vi "John's Video Viewer.vi"() -> ()   [LabVIEW 2018]
uses:
  John's Video Viewer Status STYP.ctl
  Classes/Video File/Video File.lvclass
  <vilib>/vision/Image Controls.llb/IMAQ Image.ctl
  Classes/Video Frame/Video Frame.lvclass
  Classes/Roughness Averager/Roughness Averager.lvclass
  Classes/Pointcloud/Pointcloud.lvclass
  <userlib>/Jet Engineering/JET_QSM/Code/Private/JET_QSM_InvalidOption STYP.ctl
  Classes/Video File/Video File.lvclass/Video File.ctl
  <userlib>/Jet Engineering/JET_QSM/Code/Private/JET_QSM - Add State [String API].vi
  Classes/Video File/Read Frame Data.vi
  Classes/ROIed Video Frame/ROIed Video Frame.lvclass
  C:/Users/aaron.jencks/Documents/GitHub/emerson_seed_object_detection/LabVIEW/Projects/Paul's Video Viewer/Classes/Video Frame/Video Frame.lvclass
  <vilib>/Utility/error.llb/Trim Whitespace.vi
  <vilib>/Utility/error.llb/Error Cluster From Error Code.vi
panel:
  out "width, X":i32=1280
  out "height, Y":i32=720
  out "3D Picture":refnum<vi>(3d-picture)
  out "Standard Deviation":dbl[](graph)
  in  "stop":bool
  in  "FPS":i32(slide) scale=10.0..90.0
  out "Roughness":dbl[](graph)
  out "Depth":T1(plugin-control)
  out "RGB":T1(plugin-control)
  in  "Video File":path
  out "Recent states before Error (with tick counts) 2":string="0.167 sec ago: VI Initialize\n0.167 sec ago: Window Open\n0.110 sec ago: Control Update\n0.110 sec ago: Indicator Update\n0.000 sec ago: Error Handler\r\n"
  out "error out":errorcluster
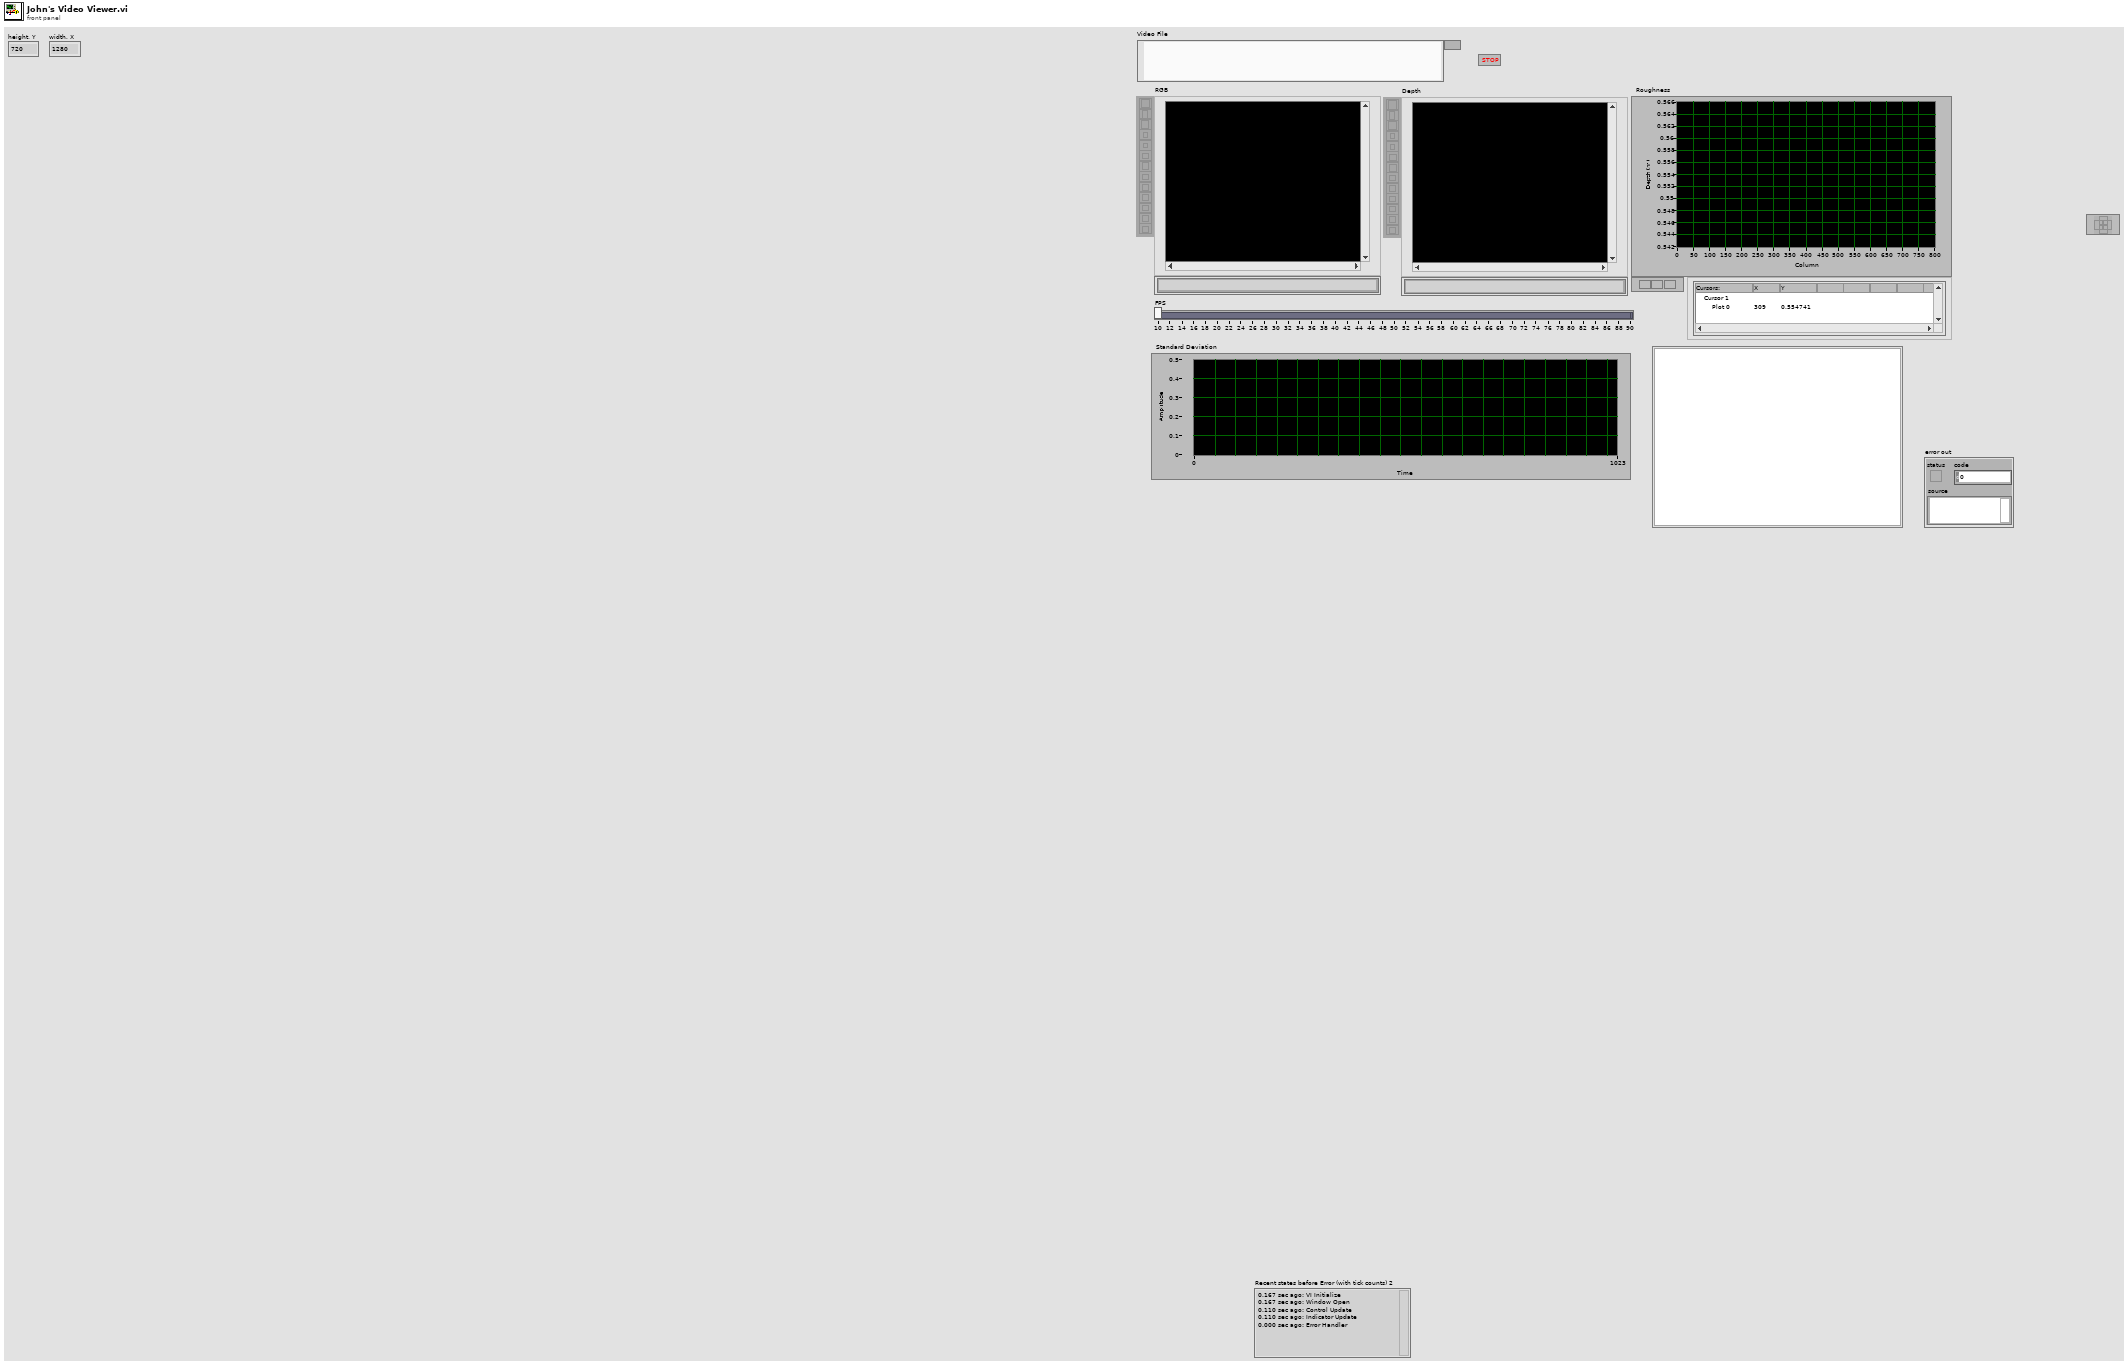
[diagram p1: front panel]
types:
  T1 = typedef "IMAQ Image.ctl" = refnum<image>
  T2 = typedef "John's Video Viewer Status STYP.ctl" = cluster{"VI":cluster{"error":errorcluster, "isExiting?":bool}, "UserLoggedIn?":bool, "RGB File":refnum<class "Video File.lvclass">, "Depth File":refnum<class "Video File.lvclass">, "RGB Image":T1, "Depth Image":T1, "RGB Frame":refnum<class "Video Frame.lvclass">, "Depth Frame":refnum<class "Video Frame.lvclass">, "FPS":i32, "History Average":refnum<queue>, "Standard Deviation":refnum<queue>, "Averager":refnum<class "Roughness Averager.lvclass">, "Pointcloud":refnum<class "Pointcloud.lvclass">}
  T3 = typedef "JET_QSM_InvalidOption STYP.ctl" = enum16{"Ignore", "Dialog", "Error"}
  T4 = typedef "JET_QSM_Refnum STYP.ctl" = cluster{"state":cluster{"queue":refnum<queue>, "idle":string, "error":string, "STOP":string}, "debug":cluster{"enabled?":bool, "queue":refnum<queue>}, "Invalid.option":T3, "QSM.Name":string}
  T5 = enum32{"invalid app kind", "Development System", "Run Time System", "Student Edition", "Embedded LabVIEW", "Evaluation", "Custom"}
  T6 = typedef "JET_QSM_Element STYP.ctl" = cluster{"state":string, "data":variant, "comment":string}
  T7 = cluster{"Width":u32, "Height":u32, "Frames Per Second":u32, "Codec":string, "Has Data":bool}
  T8 = cluster{"Global Rectangle":i32[], "Contours":cluster{"Contour Type":u32, "ROI Type":u32, "Points":i32[]}[]}
  T9 = cluster{"Normal":cluster{"Averages":cluster{"Average":dbl, "RMS":dbl, "Absolute Mean Deviation":dbl}, "Global Heuristics":cluster{"Max":dbl, "Min":dbl, "Max Peak-to-Peak":dbl}, "Skewdness":dbl, "Kurtosis":dbl, "RzDIN":dbl, "RzJIS":dbl}, "Slope Parameters":cluster{"Rdq":dbl, "Rda":dbl}, "Areal Roughness":cluster{"Peak Density":dbl}}
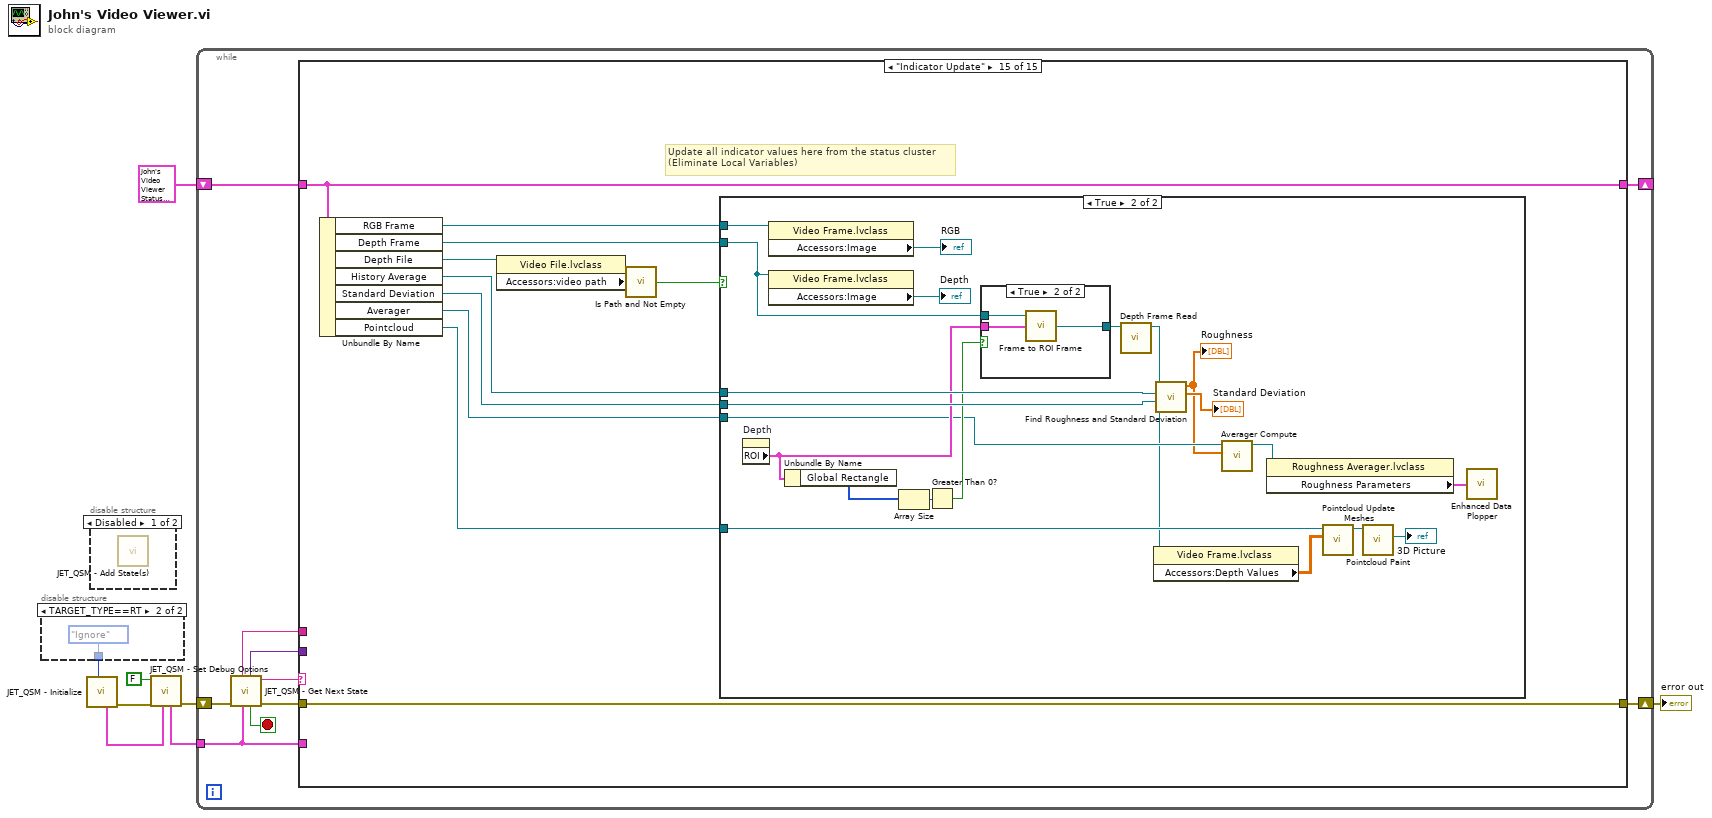
[diagram p0: block diagram]
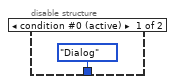
[diagram p2: hidden frame]
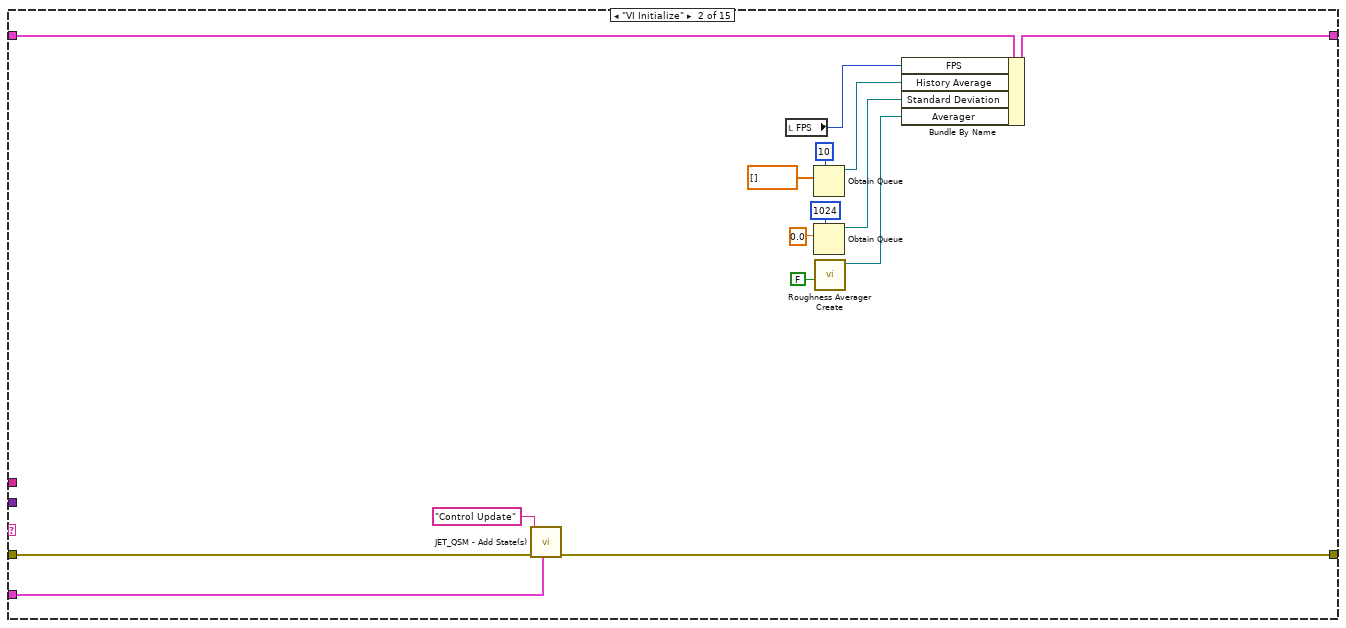
[diagram p5: hidden frame]
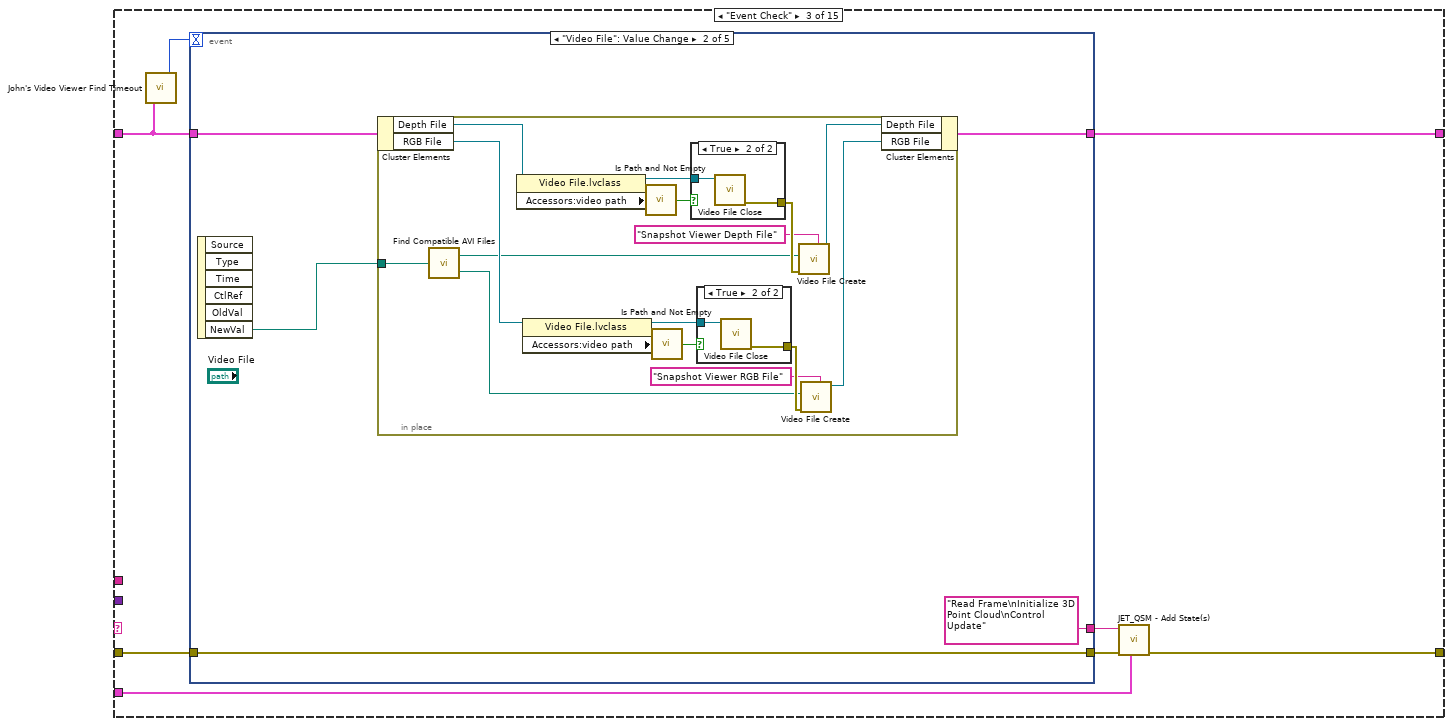
[diagram p6: hidden frame]
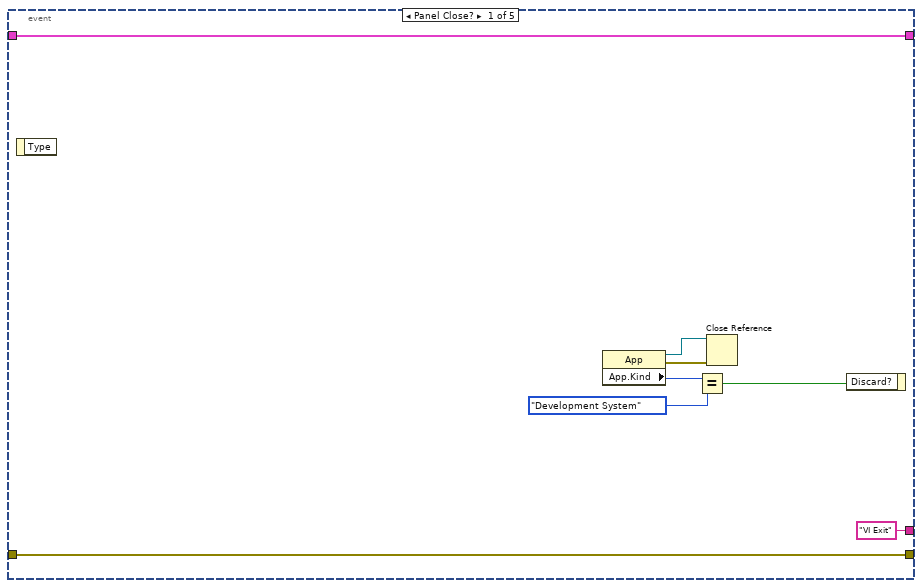
[diagram p7: hidden frame]
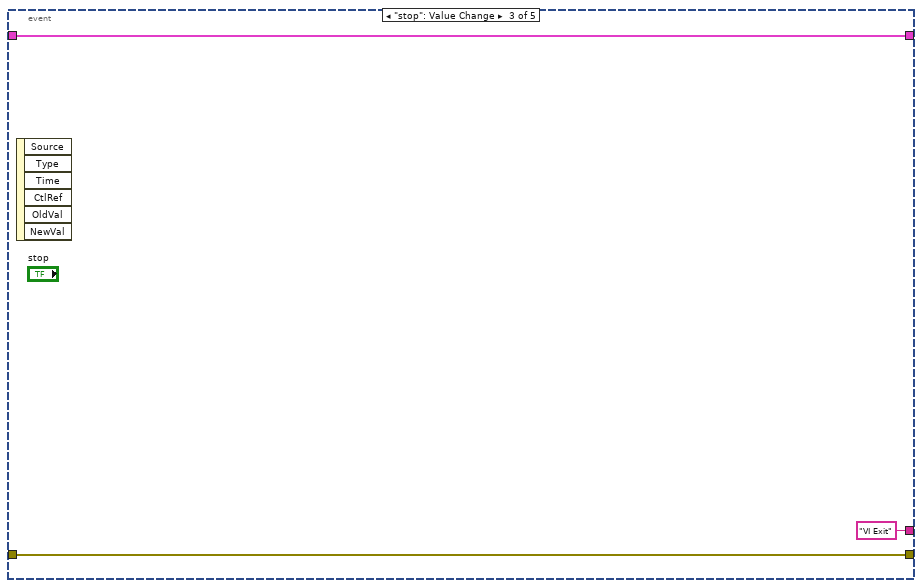
[diagram p10: hidden frame]
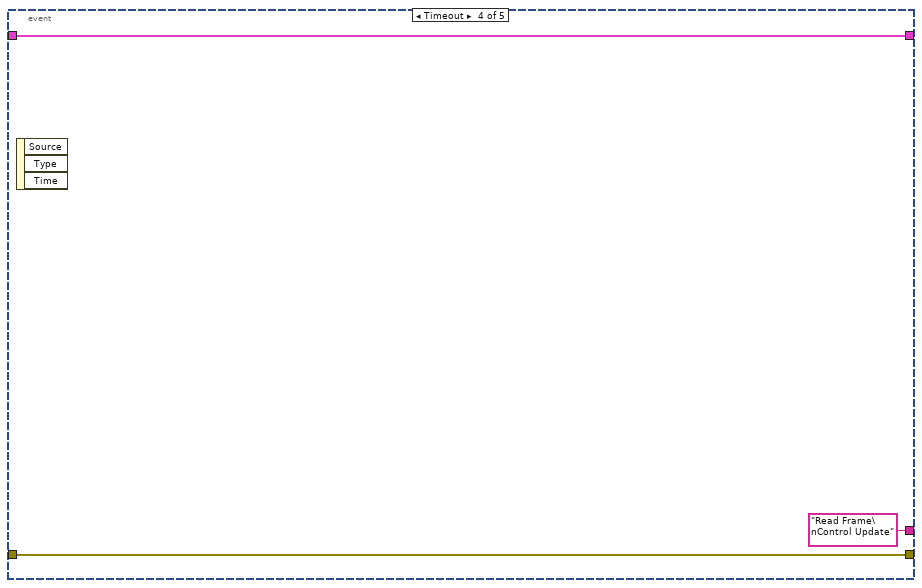
[diagram p11: hidden frame]
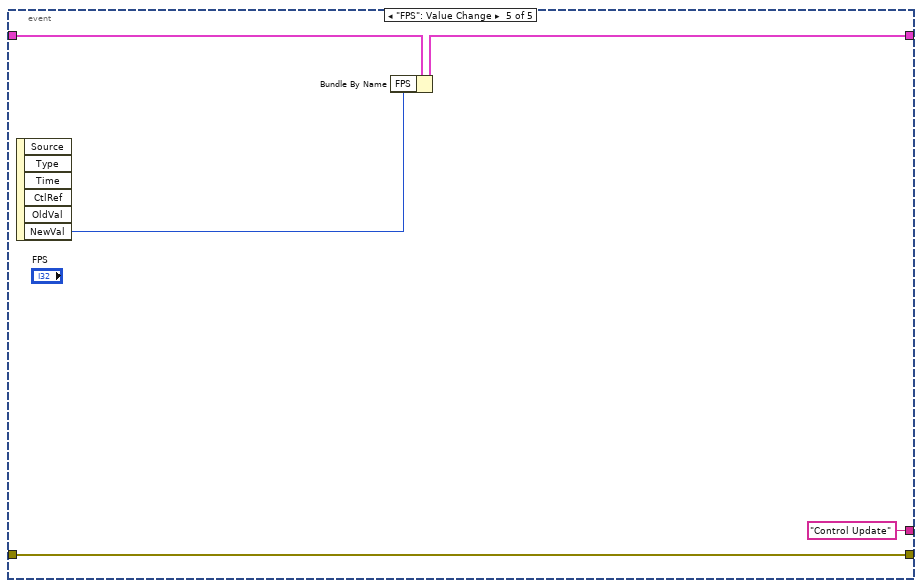
[diagram p12: hidden frame]
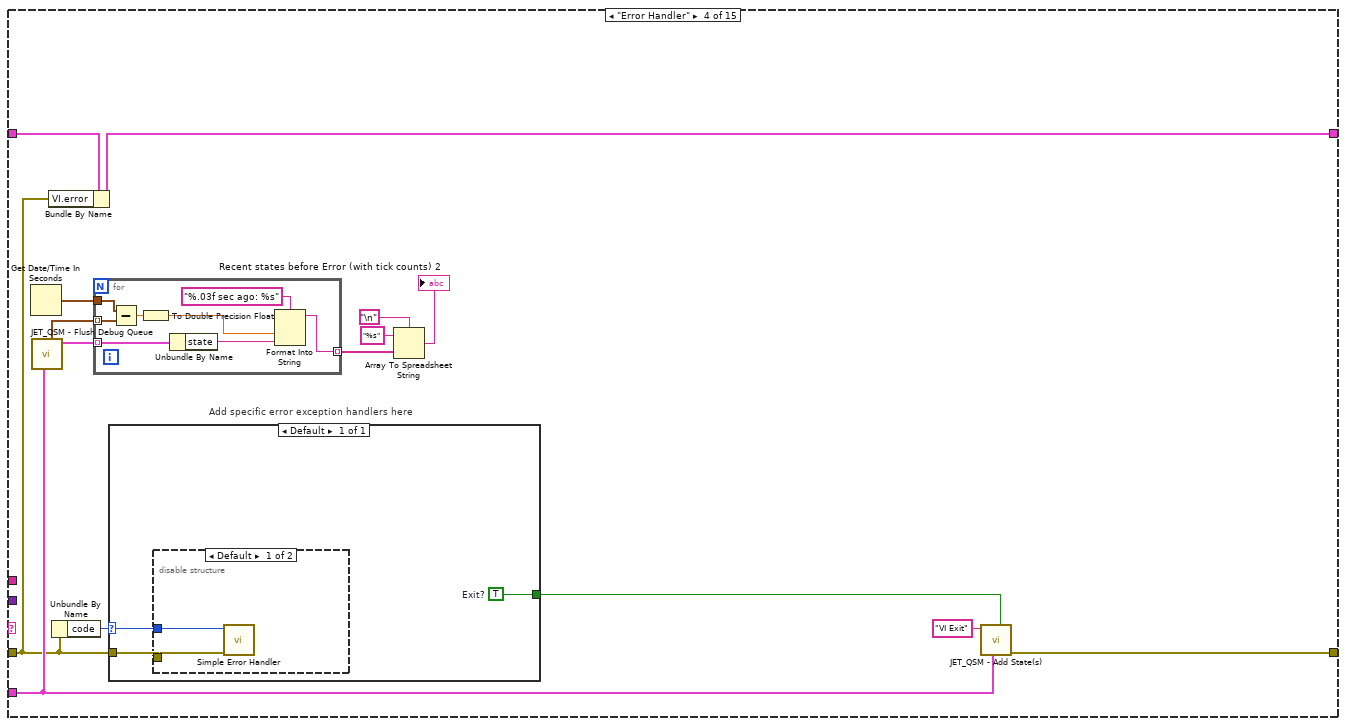
[diagram p13: hidden frame]
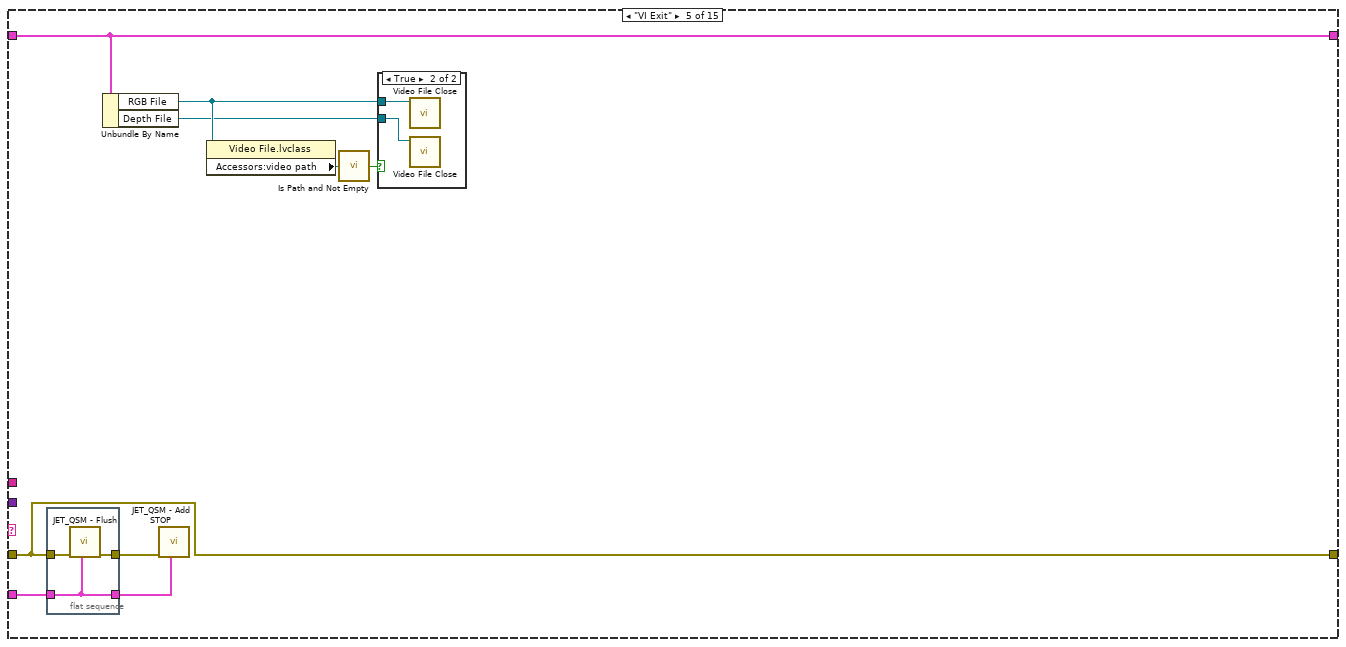
[diagram p15: hidden frame]
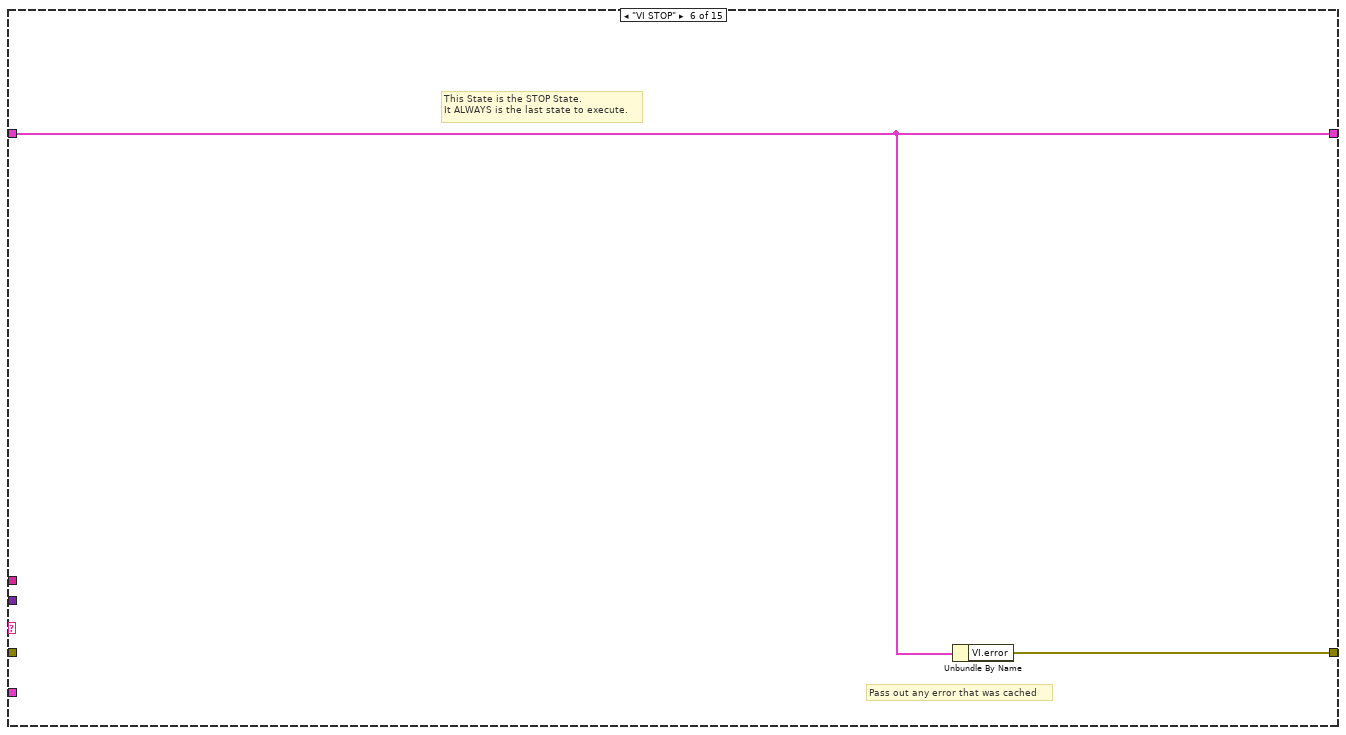
[diagram p17: hidden frame]
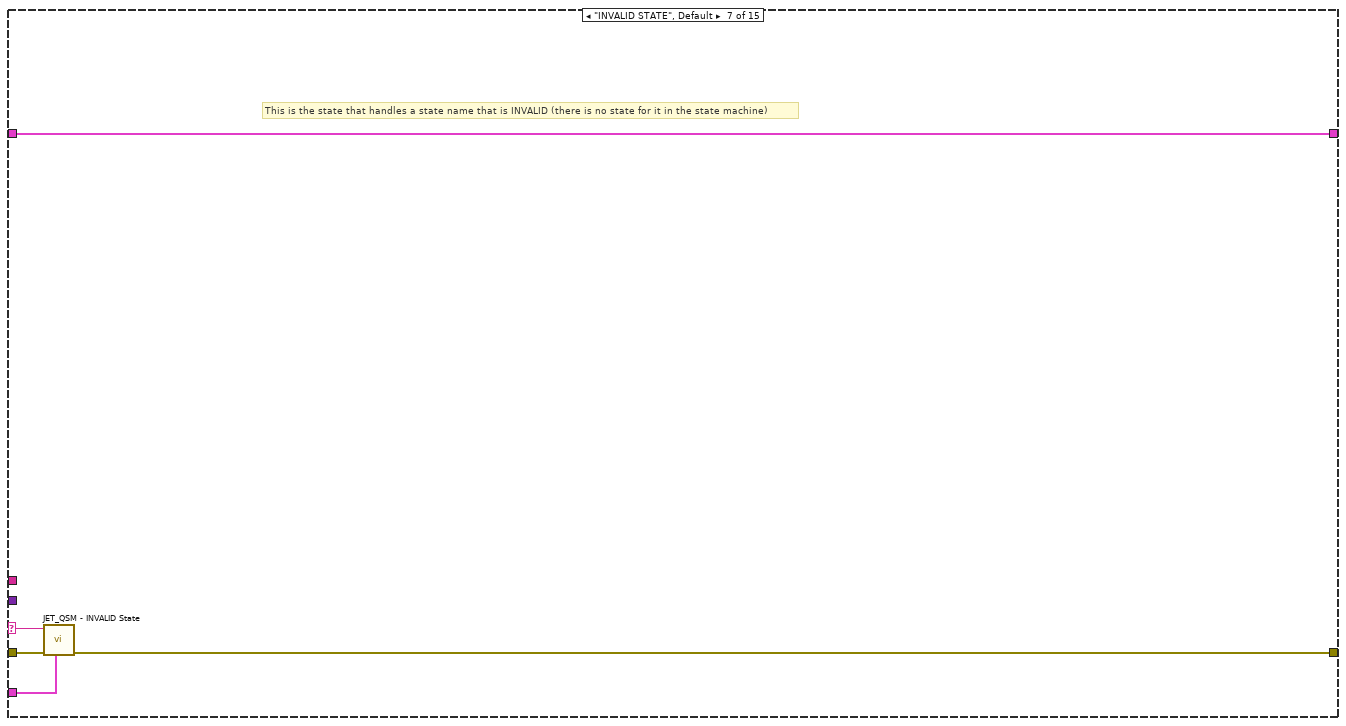
[diagram p18: hidden frame]
diagram:
  n1 = disable-structure shown="TARGET_TYPE==RT" {
    disable-tunnel: [JET_QSM_InvalidOption_STYP."Dialog" ("invalid state action (Dialog)") JET_QSM_InvalidOption_STYP."Ignore" ("invalid state action (Dialog)")] -> w8
    frame condition #0 (active) {
    }
    frame condition #1 {
    }
  }
  n2 = call <userlib>:"JET_QSM - Initialize.vi"("invalid state action (Dialog)"=w8) -> ("error out"=w1:errorcluster, "Jet_QSM refnum"=w4:T4)  [unwired: 9 in]
  n3 = disable-structure shown="Disabled" {
    frame Disabled {
      n4 = call-poly <userlib>:"JET_QSM - Add State(s).vi"() -> ()  [unwired: 11 in, 1 out]
    }
    frame Enabled {
    }
  }
  n5 = call <userlib>:"JET_QSM - Set Debug Options.vi"("Jet_QSM refnum"=w4, "error in (no error)"=w1, "debug.enabled? (F)"=FALSE) -> ("error out"=w2:errorcluster, "Jet_QSM ref"=w3:T4)  [unwired: 7 in]
  n6 = while {
    tunnel: w3 -> [w16]
    shift-right: [w14] -> _
    shift-left: T2 {"VI"={"error"={"status"=FALSE, "code"=0, "source"=""}, "isExiting?"=FALSE}, "UserLoggedIn?"=FALSE, "RGB File"=refnum, "Depth File"=refnum, "RGB Image"=refnum, "Depth Image"=refnum, "RGB Frame"=refnum, "Depth Frame"=refnum, "FPS"=0, "History Average"=refnum, "Standard Deviation"=refnum, "Averager"=refnum, "Pointcloud"=refnum} ("Status") -> [w15]
    shift-right: [w13] -> w7
    shift-left: w2 -> [w20]
    stop <- w17 stop-if-true
    n7 = call <userlib>:"JET_QSM - Get Next State.vi"("Jet_QSM refnum"=w16, "error in (no error)"=w20) -> ("error out"=w19:errorcluster, "state"=w18:string, "Stop Loop?"=w17:bool, "state data"=w12:variant, "state comment"=w11:string)  [unwired: 5 in]
    n8 = case shown="\"Indicator Update\"" w18 {
      selector: w18 -> [_ _ _ _ _ _ w137 _ _ _ _ _ _ _ _]
      tunnel: w19 -> [w21 w37 w45 w92 w127 _ w138 w140 w142 w144 w153 w156 w181 w188 w201]
      tunnel: w16 -> [_ w35 w44 w97 w125 _ w136 _ _ _ _ _ _ w189 _]
      tunnel: w15 -> [w22 w33 w38 w93 w123 w133 w139 w141 w143 w145 w150 w155 w182 w186 w200]
      tunnel: [w22 w32 w40 w91 w123 w133 w139 w141 w143 w145 w151 w154 w182 w186 w200] -> w14
      tunnel: [w21 w36 w42 w98 w127 w134 w135 w140 w142 w144 w153 w156 w181 w187 w201] -> w13
      tunnel: w12 -> [_ _ _ _ _ _ _ _ _ _ _ _ _ _ _]
      tunnel: w11 -> [_ _ _ _ _ _ _ _ _ _ _ _ _ _ _]
      frame "------ Standard States ------" {
        # "Standard States are required states for a JET_QSM State Machine\n\nTheir names may be changed; use the Initialize function to specify the new names"
        # "This is a section header; the state is never expected to execute"
      }
      frame "VI Initialize" {
        n9 = call-poly <userlib>:"JET_QSM - Add State(s).vi"("Jet_QSM refnum"=w35, "error in (no error)"=w37, "state(s)"="Control Update") -> ("error out"=w36:errorcluster)  [unwired: 8 in]
        n10 = local read "FPS"() -> (w31:i32)
        n11 = Obtain Queue(max queue size (-1, unlimited)=10, element data type=dbl[] []) -> (queue out=w29:refnum<queue>)  [unwired: 3 in, 2 out]
        n12 = Obtain Queue(max queue size (-1, unlimited)=1024, element data type=0.0) -> (queue out=w27:refnum<queue>)  [unwired: 3 in, 2 out]
        n13 = call "Roughness Averager Create.vi"("Full? (T)"=FALSE) -> ("Roughness Averager out"=w23:refnum<class "Roughness Averager.lvclass">)  [unwired: 9 in, 1 out]
        n14 = Bundle By Name(cluster=w33, "FPS"=w31, "History Average"=w29, "Standard Deviation"=w27, "Averager"=w23) -> (w32:T2)
      }
      frame "Event Check" {
        n15 = call "John's Video Viewer Find Timeout.vi"("Status"=w38) -> ("Timeout"=w39:i32)
        n16 = event shown="[1] \"Video File\": Value Change" {
          selector: _ -> [_ _ _ _ _]
          dyn-events: _ -> [_ _ _ _ _]
          timeout: w39 -> [_ _ _ _ _]
          tunnel: w45 -> [w47 w55 w81 w85 w90]
          tunnel: ["VI Exit" ("state(s)") "Read Frame\nInitialize 3D Point Cloud\nControl Update" ("state(s)") "VI Exit" ("state(s)") "Read Frame\nControl Update" ("state(s)") "Control Update" ("state(s)")] -> w43
          tunnel: [w47 w55 w81 w85 w90] -> w41
          tunnel: w38 -> [w46 w58 w82 w83 w88]
          tunnel: [w46 w57 w82 w83 w86] -> w40
          event Panel Close? {
            n17 = event-data() -> ()  [unwired: 1 in, 1 out]
            n18 = property class="App"() -> (reference out=w49:refnum<vi>, error out=w50:errorcluster, "App.Kind"=w53:T5)  [unwired: 2 in]
            n19 = Equal?(x=w53, y=T5."Development System") -> (x = y?=w51:bool)
            n20 = Close Reference(reference=w49, error in (no error)=w50) -> ()  [unwired: 1 out]
            n21 = event-data("Discard?"=w51) -> ()  [unwired: 1 in, 1 out]
          }
          event "Video File": Value Change {
            n22 = event-data() -> ("NewVal"=w56:path)  [unwired: 1 in, 5 out]
            n23 = in-place {
              in-place-border: w56 -> [w61]
              n24 = in-place-cluster #1(w58) -> ("Depth File"=w75:refnum<class "Video File.lvclass">, "RGB File"=w68:refnum<class "Video File.lvclass">)
              n25 = call "Find Compatible AVI Files.vi"("Video Path"=w61) -> ("RGB Path"=w59:path, "Depth Path"=w60:path)  [unwired: 2 in]
              n26 = property class="Video File.lvclass"(reference=w75) -> (reference out=w72:refnum<class "Video File.lvclass">, "Accessors:video path"=w74:path)  [unwired: 1 in, 1 out]
              n27 = property class="Video File.lvclass"(reference=w68) -> (reference out=w66:refnum<class "Video File.lvclass">, "Accessors:video path"=w67:path)  [unwired: 1 in, 1 out]
              n28 = call <vilib>:"Is Path and Not Empty.vi"("path"=w74) -> ("Is Path and Not Empty?"=w73:bool)  [unwired: 4 in]
              n29 = call <vilib>:"Is Path and Not Empty.vi"("path"=w67) -> ("Is Path and Not Empty?"=w65:bool)  [unwired: 4 in]
              n30 = case shown="True" w73 {
                tunnel: w72 -> [_ w79]
                tunnel: [_ w78] -> w70
                frame False {
                }
                frame True {
                  n31 = call-dynamic "Video File Close.vi"("Video File in"=w79) -> ("error out"=w78:errorcluster)  [unwired: 9 in, 1 out]
                }
              }
              n32 = case shown="True" w65 {
                tunnel: w66 -> [_ w77]
                tunnel: [_ w76] -> w64
                frame False {
                }
                frame True {
                  n33 = call-dynamic "Video File Close.vi"("Video File in"=w77) -> ("error out"=w76:errorcluster)  [unwired: 9 in, 1 out]
                }
              }
              n34 = call "Video File Create.vi"("Identifier"="Snapshot Viewer Depth File", "error in (no error)"=w70, "Video Path (\"\")"=w60) -> ("Video File out"=w71:refnum<class "Video File.lvclass">)  [unwired: 7 in, 1 out]
              n35 = call "Video File Create.vi"("Identifier"="Snapshot Viewer RGB File", "error in (no error)"=w64, "Video Path (\"\")"=w59) -> ("Video File out"=w62:refnum<class "Video File.lvclass">)  [unwired: 7 in, 1 out]
              n36 = in-place-cluster #1("Depth File"=w71, "RGB File"=w62) -> (w57:T2)
            }
          }
          event "stop": Value Change {
            n37 = event-data() -> ()  [unwired: 1 in, 6 out]
          }
          event Timeout {
            n38 = event-data() -> ()  [unwired: 1 in, 3 out]
          }
          event "FPS": Value Change {
            n39 = event-data() -> ("NewVal"=w87:i32)  [unwired: 1 in, 5 out]
            n40 = Bundle By Name(cluster=w88, "FPS"=w87) -> (w86:T2)
          }
        }
        n41 = call-poly <userlib>:"JET_QSM - Add State(s).vi"("Jet_QSM refnum"=w44, "error in (no error)"=w41, "state(s)"=w43) -> ("error out"=w42:errorcluster)  [unwired: 8 in]
      }
      frame "Error Handler" {
        # "Add specific error exception handlers here"
        n42 = Get Date/Time In Seconds() -> (seconds since 1Jan1904=w101:timestamp)
        n43 = call <userlib>:"JET_QSM - Flush Debug Queue.vi"("Jet_QSM refnum"=w97) -> ("QSM Elements"=w99:T6[], "Timestamps"=w100:timestamp[])  [unwired: 8 in, 1 out]
        n44 = Bundle By Name(cluster=w93, "VI.error"=w92) -> (w91:T2)
        n45 = Unbundle By Name(w92) -> ("code"=w94:i32)
        n46 = for {
          tunnel: w99 -> [w113] mode=indexing
          tunnel: [w111] -> w103 mode=indexing
          tunnel: w101 -> [w108]
          tunnel: w100 -> [w109] mode=indexing
          n47 = Subtract(x=w108, y=w109) -> (x-y=w107:dbl)
          n48 = To Double Precision Float(number=w107) -> (double precision float=w106:dbl)
          n49 = Unbundle By Name(w113) -> ("state"=w112:string)
          n50 = Format Into String(format string="%.03f sec ago: %s", w106, w112) -> (resulting string=w111:string)  [unwired: 2 in, 1 out]
        }
        n51 = case shown="Default" w94 {
          selector: w94 -> [w115]
          tunnel: [w116] -> w95
          tunnel: w92 -> [w114]
          frame Default {
            w116 = TRUE  # Exit?
            n52 = disable-structure shown="Default" {
              disable-tunnel: w115 -> [w118 _]
              disable-tunnel: w114 -> [w117 _]
              frame condition #0 (active) {
                n53 = call <vilib>:"Simple Error Handler.vi"("error code (no error:0)"=w118, "error in (no error)"=w117) -> ()  [unwired: 3 in, 5 out]
              }
              frame condition #1 {
              }
            }
          }
        }
        n54 = Array To Spreadsheet String(delimiter (Tab)="\n", array=w103, 3:"%s" ("format string")) -> (spreadsheet string=→"Recent states before Error (with tick counts) 2":string)
        n55 = call-poly <userlib>:"JET_QSM - Add State(s).vi"("act? (T)"=w95, "Jet_QSM refnum"=w97, "state(s)"="VI Exit") -> ("error out"=w98:errorcluster)  [unwired: 8 in]
      }
      frame "VI Exit" {
        n56 = flat-sequence {
          tunnel: w127 -> [w132]
          tunnel: [w131] -> w126
          tunnel: w125 -> [w130]
          tunnel: [w130] -> w124
          frame #0 {
            n57 = call <userlib>:"JET_QSM - Flush.vi"("Jet_QSM ref"=w130, "error in (no error)"=w132) -> ("error out"=w131:errorcluster)  [unwired: 8 in, 1 out]
          }
        }
        n58 = Unbundle By Name(w123) -> ("RGB File"=w120:refnum<class "Video File.lvclass">, "Depth File"=w119:refnum<class "Video File.lvclass">)
        n59 = call <userlib>:"JET_QSM - Add STOP.vi"("Jet_QSM refnum"=w124, "error in (no error)"=w126) -> ()  [unwired: 9 in, 1 out]
        n60 = property class="Video File.lvclass"(reference=w120) -> ("Accessors:video path"=w122:path)  [unwired: 1 in, 2 out]
        n61 = call <vilib>:"Is Path and Not Empty.vi"("path"=w122) -> ("Is Path and Not Empty?"=w121:bool)  [unwired: 4 in]
        n62 = case shown="True" w121 {
          tunnel: w120 -> [_ w129]
          tunnel: w119 -> [_ w128]
          frame False {
          }
          frame True {
            n63 = call-dynamic "Video File Close.vi"("Video File in"=w129) -> ()  [unwired: 9 in, 2 out]
            n64 = call-dynamic "Video File Close.vi"("Video File in"=w128) -> ()  [unwired: 9 in, 2 out]
          }
        }
      }
      frame "VI STOP" {
        # "Pass out any error that was cached"
        # "This State is the STOP State.\nIt ALWAYS is the last state to execute."
        n65 = Unbundle By Name(w133) -> ("VI.error"=w134:errorcluster)
      }
      frame "INVALID STATE", Default {
        # "This is the state that handles a state name that is INVALID (there is no state for it in the state machine)"
        n66 = call <userlib>:"JET_QSM - INVALID State.vi"("Jet_QSM refnum"=w136, "error in (no error)"=w138, "state"=w137) -> ("error out"=w135:errorcluster)  [unwired: 8 in]
      }
      frame "------ Menu Commands ------" {
        # "This is a section header; the state is never expected to execute"
      }
      frame "------ Events  ------" {
        # "This is a section header; the state is never expected to execute"
      }
      frame "------ Actions  ------" {
        # "This is a section header; the state is never expected to execute"
      }
      frame "Initialize 3D Point Cloud" {
        n67 = Unbundle By Name(w150) -> ("Depth File"=w149:refnum<class "Video File.lvclass">)
        n68 = property class="Video File.lvclass"(reference=w149) -> ("Accessors:Frame Data"=w148:T7)  [unwired: 1 in, 2 out]
        n69 = Unbundle By Name(w148) -> ("Width"=w146:u32, "Height"=w147:u32)
        n70 = call "Pointcloud Create.vi"("Width"=w146, "Height"=w147) -> ("Pointcloud out"=w152:refnum<class "Pointcloud.lvclass">)  [unwired: 8 in, 1 out]
        n71 = Bundle By Name(cluster=w150, "Pointcloud"=w152) -> (w151:T2)
      }
      frame "Read Frame" {
        n72 = in-place {
          n73 = in-place-cluster #2(w155) -> ("RGB File"=w170:refnum<class "Video File.lvclass">, "Depth File"=w169:refnum<class "Video File.lvclass">, "RGB Image"=w160:T1, "Depth Image"=w159:T1)  [unwired: 2 out]
          n74 = property class="Video File.lvclass"(reference=w170) -> (reference out=w165:refnum<class "Video File.lvclass">, "Accessors:video path"=w168:path)  [unwired: 1 in, 1 out]
          n75 = property class="Video File.lvclass"(reference=w169) -> (reference out=w163:refnum<class "Video File.lvclass">, "Accessors:video path"=w167:path)  [unwired: 1 in, 1 out]
          n76 = call <vilib>:"Is Path and Not Empty.vi"("path"=w168) -> ("Is Path and Not Empty?"=w166:bool)  [unwired: 4 in]
          n77 = call <vilib>:"Is Path and Not Empty.vi"("path"=w167) -> ("Is Path and Not Empty?"=w162:bool)  [unwired: 4 in]
          n78 = case shown="True" w166 {
            tunnel: w165 -> [w176 w180]
            tunnel: w160 -> [_ w179]
            tunnel: [w176 w178] -> w164
            tunnel: [_ w177] -> w158
            frame False {
            }
            frame True {
              n79 = call-dynamic "Video File Frame Read.vi"("Image Dst"=w179, "Video File in"=w180) -> ("Video Frame out"=w177:refnum<class "Video Frame.lvclass">, "Video File out"=w178:refnum<class "Video File.lvclass">)  [unwired: 5 in, 3 out]
            }
          }
          n80 = case shown="True" w162 {
            tunnel: w163 -> [w171 w175]
            tunnel: w159 -> [_ w174]
            tunnel: [w171 w173] -> w161
            tunnel: [_ w172] -> w157
            frame False {
            }
            frame True {
              n81 = call-dynamic "Video File Frame Read.vi"("Image Dst"=w174, "Video File in"=w175) -> ("Video Frame out"=w172:refnum<class "Video Frame.lvclass">, "Video File out"=w173:refnum<class "Video File.lvclass">)  [unwired: 5 in, 3 out]
            }
          }
          n82 = in-place-cluster #2("RGB File"=w164, "Depth File"=w161, "RGB Image"=w160, "Depth Image"=w159, "RGB Frame"=w158, "Depth Frame"=w157) -> (w154:T2)
        }
      }
      frame "------ Window and Panel Control ------" {
        # "This is a section header; the state is never expected to execute"
      }
      frame "Control Update" {
        # "Update all control properties here from the status cluster\n(Consolidate/reduce property nodes)"
        n83 = Unbundle By Name(w186) -> ("Depth File"=w185:refnum<class "Video File.lvclass">, "FPS"=w183:i32)
        n84 = property class="Video File.lvclass"(reference=w185) -> ("Accessors:video path"=w184:path)  [unwired: 1 in, 2 out]
        n85 = local write "Video File"(w184) -> ()
        n86 = local write "FPS"(w183) -> ()
        n87 = call-poly <userlib>:"JET_QSM - Add State(s).vi"("Jet_QSM refnum"=w189, "error in (no error)"=w188, "state(s)"="Indicator Update") -> ("error out"=w187:errorcluster)  [unwired: 8 in]
      }
      frame "Indicator Update" {
        # "Update all indicator values here from the status cluster\n(Eliminate Local Variables)"
        n88 = Unbundle By Name(w200) -> ("RGB Frame"=w199:refnum<class "Video Frame.lvclass">, "Depth Frame"=w198:refnum<class "Video Frame.lvclass">, "Depth File"=w197:refnum<class "Video File.lvclass">, "History Average"=w194:refnum<queue>, "Standard Deviation"=w193:refnum<queue>, "Averager"=w192:refnum<class "Roughness Averager.lvclass">, "Pointcloud"=w191:refnum<class "Pointcloud.lvclass">)
        n89 = property class="Video File.lvclass"(reference=w197) -> ("Accessors:video path"=w196:path)  [unwired: 1 in, 2 out]
        n90 = call <vilib>:"Is Path and Not Empty.vi"("path"=w196) -> ("Is Path and Not Empty?"=w195:bool)  [unwired: 4 in]
        n91 = case shown="True" w195 {
          tunnel: w199 -> [_ w222]
          tunnel: w198 -> [_ w212]
          tunnel: w194 -> [_ w219]
          tunnel: w193 -> [_ w218]
          tunnel: w192 -> [_ w210]
          tunnel: w191 -> [_ w206]
          frame False {
          }
          frame True {
            n92 = property on="Depth" class="ImageControl"() -> ("ROI"=w213:T8)  [unwired: 2 in, 2 out]
            n93 = property class="Video Frame.lvclass"(reference=w222) -> ("Accessors:Image"=→"RGB":T1)  [unwired: 1 in, 2 out]
            n94 = property class="Video Frame.lvclass"(reference=w212) -> ("Accessors:Image"=→"Depth":T1)  [unwired: 1 in, 2 out]
            n95 = Unbundle By Name(w213) -> ("Global Rectangle"=w216:i32[])
            n96 = Array Size(array=w216) -> (size(s)=w215:i32)
            n97 = Greater Than 0?(x=w215) -> (x > 0?=w214:bool)
            n98 = case shown="True" w214 {
              tunnel: w212 -> [w223 w226]
              tunnel: w213 -> [_ w225]
              tunnel: [w223 w224] -> w211
              frame False {
              }
              frame True {
                n99 = call "Frame to ROI Frame.vi"("ROI Descriptor"=w225, "Video Frame"=w226) -> ("ROIed Video Frame"=w224:refnum<class "ROIed Video Frame.lvclass">)  [unwired: 1 in]
              }
            }
            n100 = call-dynamic "Depth Frame Read.vi"("Video Frame in"=w211) -> ("Video Frame out"=w205:refnum<class "Video Frame.lvclass">)  [unwired: 6 in, 4 out]
            n101 = property class="Video Frame.lvclass"(reference=w205) -> ("Accessors:Depth Values"=w204:dbl[][])  [unwired: 1 in, 2 out]
            n102 = call "Find Roughness and Standard Deviation.vi"("Standard Deviation"=w218, "History Average"=w219, "Video Frame in"=w205) -> ("elements"=→"Standard Deviation":dbl[], "Column Averages"=w209:dbl[])  [unwired: 7 in]
            "Roughness" <- w209
            n103 = call-dynamic "Averager Compute.vi"("Data"=w209, "Roughness Averager in"=w210) -> ("Roughness Averager out"=w208:refnum<class "Roughness Averager.lvclass">)  [unwired: 8 in, 1 out]
            n104 = property class="Roughness Averager.lvclass"(reference=w208) -> ("Roughness Parameters"=w207:T9)  [unwired: 1 in, 2 out]
            n105 = call-dynamic "Pointcloud Update Meshes.vi"("2D Map"=w204, "Pointcloud in"=w206) -> ("Pointcloud out"=w203:refnum<class "Pointcloud.lvclass">)  [unwired: 8 in, 1 out]
            n106 = call-dynamic "Pointcloud Paint.vi"("Pointcloud in"=w203) -> ("Pointcloud"=→"3D Picture":refnum<vi>)  [unwired: 8 in, 2 out]
            n107 = call "Enhanced Data Plopper.vi"("Roughness"=w207) -> ()
          }
        }
      }
    }
  }
  "error out" <- w7
